vi "WS1021 CS Beam VCmin.vi"(7 "Reg":string[](array[string])=["43", "42", "43", "43", "43", "43", "43", "43", "42", "42", "42", "42", "42", "42"], 8 "Error In":errorcluster, 10 "Cmd Bit":string[](array[string])=["40", "40", "20", "01", "02", "04", "08", "10", "01", "02", "04", "08", "10", "20"], 11 "Driver Name":string[](array[string])=["FB1", "FB2", "FB3", "TB1", "TB2", "TB3", "TB4", "TB5", "TB6", "TB7", "TB8", "TB9", "TB10", "TB11"]) -> (0 "Error Out":errorcluster, 2 "Beam Cmd OFF":string[](array[string]), 3 "Beam Cmd":string[](array[string]), 5 "CS_Driver Name":string[](array[string]))   [LabVIEW 2017]
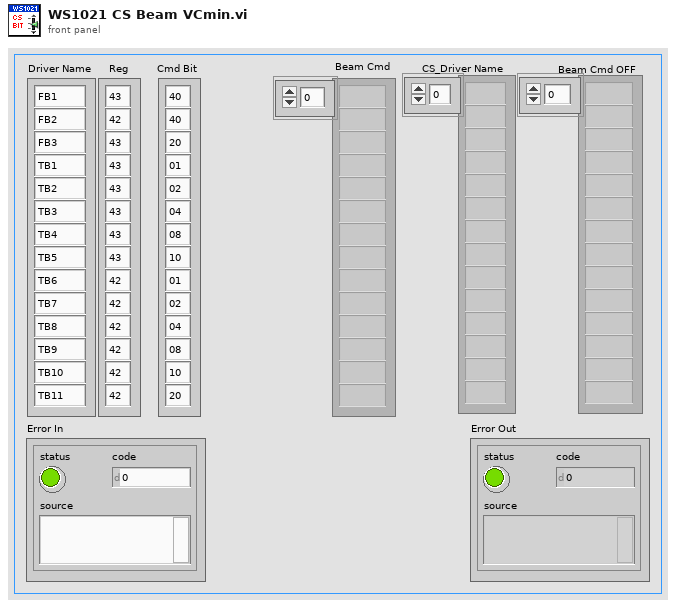
[diagram p1: front panel]
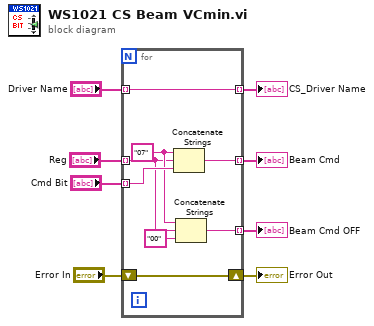
[diagram p0: block diagram]
diagram:
  n1 = for {
    tunnel: "Driver Name" -> [w13] mode=indexing
    tunnel: "Cmd Bit" -> [w16] mode=indexing
    tunnel: "Reg" -> [w11] mode=indexing
    tunnel: [w15] -> w5 mode=indexing
    shift-right: [w14] -> w3
    shift-left: "Error In" -> [w14]
    tunnel: [w13] -> w2 mode=indexing
    tunnel: [w9] -> w1 mode=indexing
    w12 = "07" ("string")
    n2 = Concatenate Strings(w12, w11, w16) -> (w15:string)
    n3 = Concatenate Strings(w12, w11, "00" ("string")) -> (w9:string)
  }
  "Beam Cmd" <- w5
  "Error Out" <- w3
  "CS_Driver Name" <- w2
  "Beam Cmd OFF" <- w1
